vi "加密解密字符串应用举例（XOR 数组）.vi"() -> ()   [LabVIEW 2012]
panel:
  in  "密钥字符串":string
  out "加密后字符串":string
  out "输出字符串":string
  in  "输入字符串":string
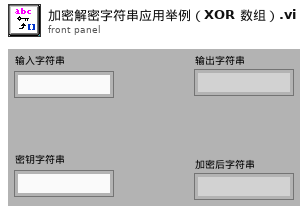
[diagram p1: front panel]
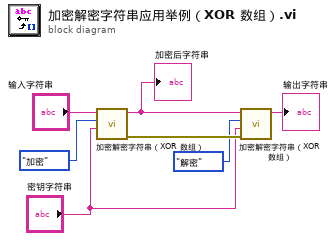
[diagram p0: block diagram]
diagram:
  n1 = call "加密解密字符串（XOR 数组）.vi"("密钥"="密钥字符串", "模式"=enum16{"加密", "解密"}."加密", "输入字符串"="输入字符串") -> ("error out"=w4:errorcluster, "输出字符串"=w5:string)  [unwired: 7 in]
  "加密后字符串" <- w5
  n2 = call "加密解密字符串（XOR 数组）.vi"("error in (no error)"=w4, "密钥"="密钥字符串", "模式"=enum16{"加密", "解密"}."解密", "输入字符串"=w5) -> ("输出字符串"=→"输出字符串":string)  [unwired: 6 in, 1 out]
